vi "AVI Video-Clear file paths.vi"(8 "error in (no error)":errorcluster) -> (0 "error out":errorcluster)   [LabVIEW 2017]
uses:
  Typedefs/Channel Selector.ctl
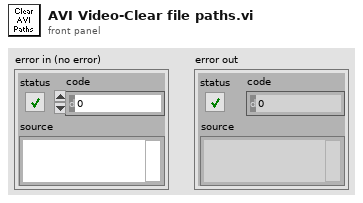
[diagram p1: front panel]
types:
  T1 = typedef "Channel Selector.ctl" = enum16{"Red Channel", "Green Channel", "Blended"}
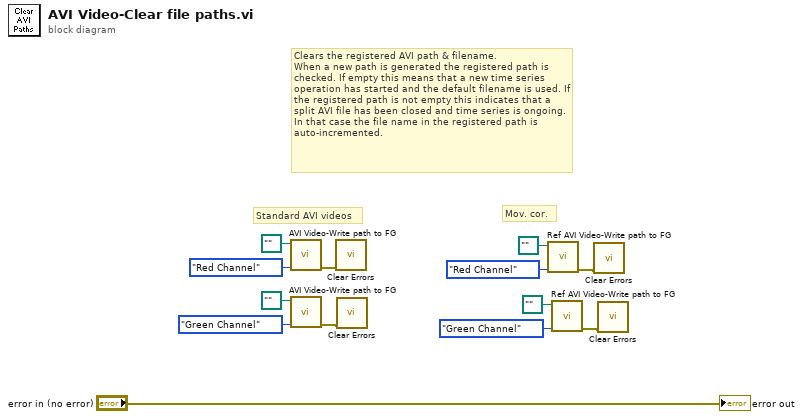
[diagram p0: block diagram]
diagram:
  # "Standard AVI videos"
  # "Mov. cor."
  # "Clears the registered AVI path & filename.\nWhen a new path is generated the registered path is checked. If empty this means that a new time series operation has started and the default filename is used. If the registered path is not empty this indicates that a split AVI file has been closed and time series is ongoing. In that case the file name in the registered path is auto-incremented."
  n1 = call "AVI Video-Write path to FG.vi"("Channel"=Channel_Selector."Red Channel", "AVI2 path"=path "") -> ("error out"=w8:errorcluster)  [unwired: 9 in]
  n2 = call "AVI Video-Write path to FG.vi"("Channel"=Channel_Selector."Green Channel", "AVI2 path"=path "") -> ("error out"=w7:errorcluster)  [unwired: 9 in]
  n3 = call <vilib>:"Clear Errors.vi"("error in (no error)"=w8) -> ()  [unwired: 5 in, 2 out]
  n4 = call <vilib>:"Clear Errors.vi"("error in (no error)"=w7) -> ()  [unwired: 5 in, 2 out]
  n5 = call "Ref AVI Video-Write path to FG.vi"("Channel"=Channel_Selector."Red Channel", "AVI2 path"=path "") -> ("error out"=w1:errorcluster)  [unwired: 9 in]
  n6 = call "Ref AVI Video-Write path to FG.vi"("Channel"=Channel_Selector."Green Channel", "AVI2 path"=path "") -> ("error out"=w6:errorcluster)  [unwired: 9 in]
  n7 = call <vilib>:"Clear Errors.vi"("error in (no error)"=w1) -> ()  [unwired: 5 in, 2 out]
  n8 = call <vilib>:"Clear Errors.vi"("error in (no error)"=w6) -> ()  [unwired: 5 in, 2 out]
  "error out" <- "error in (no error)"
